vi "AG34405 Measure DC Current.vi"(0 "VISA resource name":refnum<visa-resource-name>, 5 "Range (6:Auto)":T2(ring)=enum."Auto", 9 "Resolution (5:Default)":T1(ring)=enum."Default", 11 "error in (no error)":errorcluster, 12 "Byte Count (1024 bytes)":i32=1024, 13 "Timeout (40 sec)":i32=40000) -> (4 "VISA resource name out":refnum<visa-resource-name>, 6 "Output Array":dbl[](array[numeric]) format="%.2e", 15 "error out":errorcluster)   [LabVIEW 2018]
doc: "First, this command resets all DC current measurement parameters and trigger parameters to their default values. Then, it configures the meter for DC current measurements and immediately triggers a measurement. The results are sent directly to the instrument output buffer."
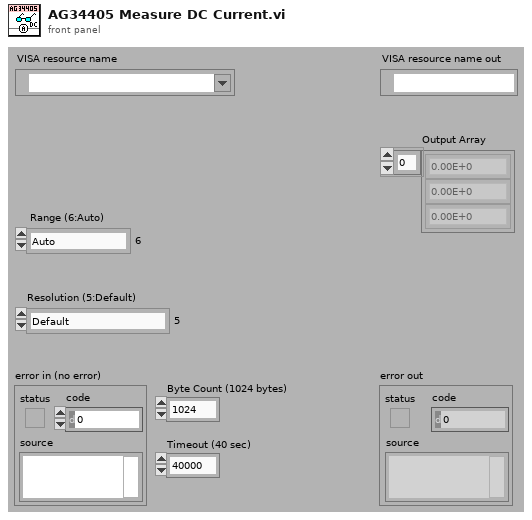
[diagram p1: front panel]
types:
  T1 = enum16{"4 1/2", "5 1/2", "6 1/2", "Least", "Highest", "Default"}
  T2 = enum16{"100 uA", "1 mA", "10 mA", "100 mA", "1 A", "3 A", "Auto", "Minimum", "Maximum", "Default"}
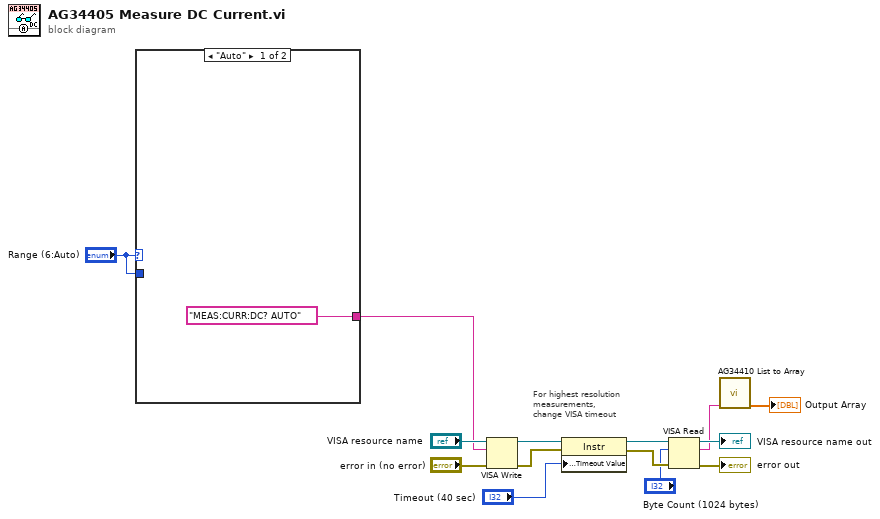
[diagram p0: block diagram]
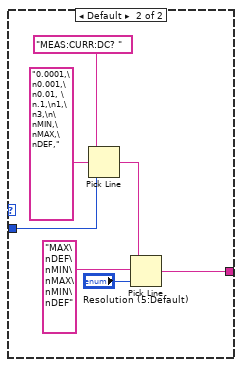
[diagram p2: hidden frame]
diagram:
  # "For highest resolution\nmeasurements, \nchange VISA timeout"
  n1 = case shown="\"Auto\"" "Range (6:Auto)" {
    tunnel: "Range (6:Auto)" -> [_ w19]
    tunnel: ["MEAS:CURR:DC? AUTO" w17] -> w1
    frame "Auto" {
    }
    frame Default {
      n2 = Pick Line(string ("")="MEAS:CURR:DC? ", multi-line string="0.0001,\n0.001,\n0.01, \n.1,\n1,\n3,\n\nMIN,\nMAX,\nDEF,", line index=w19) -> (output string=w18:string)
      n3 = Pick Line(string ("")=w18, multi-line string="MAX\nDEF\nMIN\nMAX\nMIN\nDEF", line index="Resolution (5:Default)") -> (output string=w17:string)
    }
  }
  n4 = VISA Write(VISA resource name="VISA resource name", write buffer=w1, error in (no error)="error in (no error)") -> (VISA resource name out=w7:refnum<visa-resource-name>, error out=w5:errorcluster)  [unwired: 1 out]
  n5 = property class="Instr"(reference=w7, error in=w5, "General Settings:Timeout Value"="Timeout (40 sec)") -> (reference out=w6:refnum<visa-resource-name>, error out=w14:errorcluster)
  n6 = VISA Read(VISA resource name=w6, byte count="Byte Count (1024 bytes)", error in (no error)=w14) -> (VISA resource name out=→"VISA resource name out":refnum<visa-resource-name>, read buffer=w2:string, error out=→"error out":errorcluster)  [unwired: 1 out]
  n7 = call <instrlib>:"AG34410 List to Array.vi"("List"=w2) -> ("Output Number Array"=→"Output Array":dbl[])  [unwired: 3 in, 3 out]
